vi "Get Tunnel Diagrams.vi"(8 "error in":errorcluster, 11 "Tunnel in":refnum<vi>) -> (0 "error out":errorcluster, 1 "Inner Diagram found?":bool, 2 "Inner Diagram":refnum<vi>, 3 "Outer Diagram":refnum<vi>, 4 "Inner Terminal":refnum<vi>, 5 "Outer Terminal":refnum<vi>)   [LabVIEW 2023]
doc: "Returns the outer diagram and inner diagram references for a tunnel. the inner will be the currently displayed frame on a multi-frame structure, suce as an event or case structure."
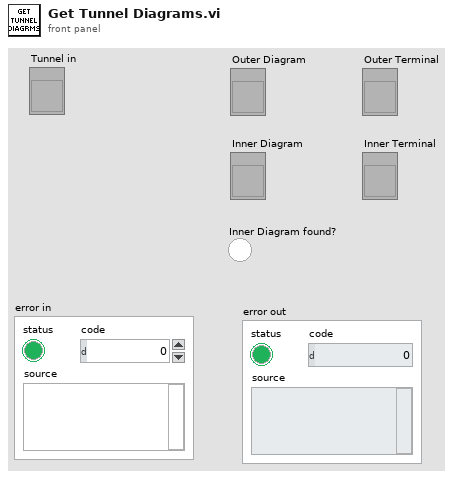
[diagram p1: front panel]
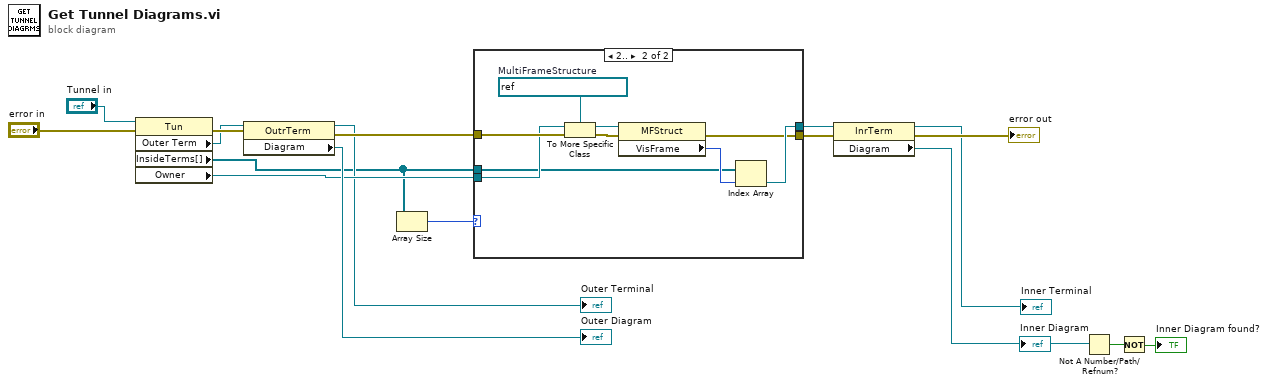
[diagram p0: block diagram]
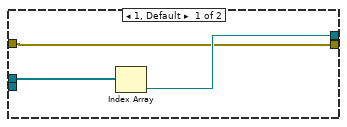
[diagram p2: hidden frame]
diagram:
  n1 = property class="Tun"(reference="Tunnel in", error in="error in") -> (error out=w7:errorcluster, "Outer Term"=w5:refnum<vi>, "InsideTerms[]"=w2:refnum<vi>[], "Owner"=w6:refnum<vi>)  [unwired: 1 out]
  n2 = property class="OutrTerm"(reference=w5, error in=w7) -> (reference out=→"Outer Terminal":refnum<vi>, error out=w13:errorcluster, "Diagram"=→"Outer Diagram":refnum<vi>)
  n3 = Array Size(array=w2) -> (size(s)=w1:i32)
  n4 = case shown="2.." w1 {
    tunnel: w13 -> [w18 w29]
    tunnel: [w19 w28] -> w9
    tunnel: [w18 w23] -> w8
    tunnel: w6 -> [_ w22]
    tunnel: w2 -> [w20 w21]
    frame 1, Default {
      n5 = Index Array(array=w20) -> (element=w19:refnum<vi>)  [unwired: 1 in]
    }
    frame 2.. {
      w26 = refnum<vi> refnum  # MultiFrameStructure
      n6 = To More Specific Class(target class=w26, reference=w22, error in=w29) -> (specific class reference=w27:refnum<vi>, error out=w25:errorcluster)
      n7 = property class="MFStruct"(reference=w27, error in=w25) -> (error out=w23:errorcluster, "VisFrame"=w24:u32)  [unwired: 1 out]
      n8 = Index Array(array=w21, index=w24) -> (element=w28:refnum<vi>)
    }
  }
  n9 = property class="InrTerm"(reference=w9, error in=w8) -> (reference out=→"Inner Terminal":refnum<vi>, error out=→"error out":errorcluster, "Diagram"=w15:refnum<vi>)
  "Inner Diagram" <- w15
  n10 = Not A Number/Path/Refnum?(number/path/refnum=w15) -> (NaN/Path/Refnum?=w14:bool)
  n11 = Not(x=w14) -> (.not. x?=→"Inner Diagram found?":bool)
